vi "Global.vi"() -> ()   [LabVIEW 2015]
uses:
  network/network.lvclass
panel:
  out "ADODB._Connection Out":refnum<k7>
  in  "network.lvclass":refnum<class "network.lvclass">
  in  "远程地址":refnum<visa-resource-name>
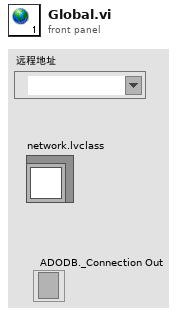
[diagram p1: front panel]
diagram:
